vi "mod_Quantize BPSK symbols.vi"(0 "input data":dbl[](array[numeric]), 5 "quantization bits":i32=1, 11 "error in (no error)":errorcluster) -> (4 "output data":i32[](array[numeric]), 15 "error out":errorcluster)   [LabVIEW 2020, in "niDMT.lvlib"]
uses:
  <vilib>/addons/Modulation/niDMT.lvlib
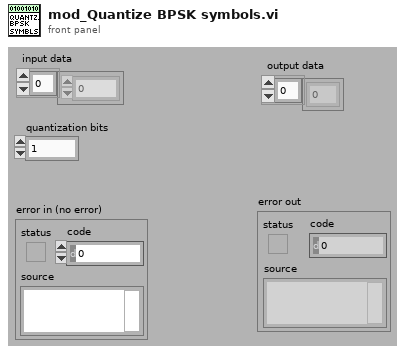
[diagram p1: front panel]
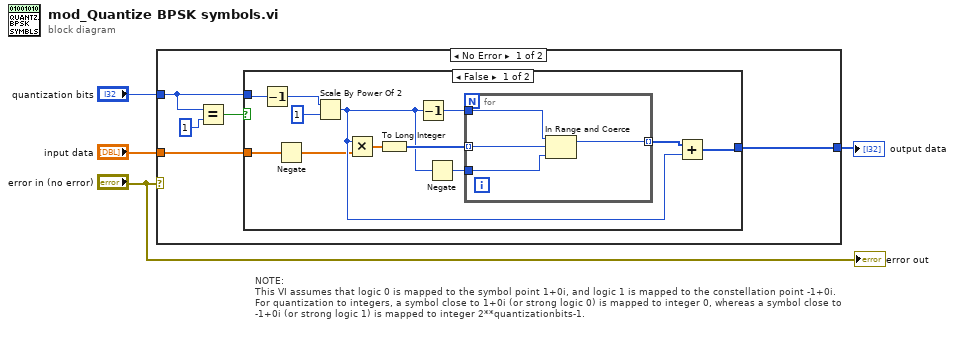
[diagram p0: block diagram]
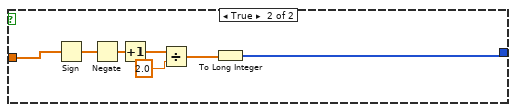
[diagram p2: hidden frame]
diagram:
  # "NOTE: \nThis VI assumes that logic 0 is mapped to the symbol point 1+0i, and logic 1 is mapped to the constellation point -1+0i.\nFor quantization to integers, a symbol close to 1+0i (or strong logic 0) is mapped to integer 0, whereas a symbol close to\n-1+0i (or strong logic 1) is mapped to integer 2**quantizationbits-1."
  n1 = case shown="No Error" "error in (no error)" {
    tunnel: "quantization bits" -> [w7 _]
    tunnel: "input data" -> [w9 _]
    tunnel: [w8 _] -> w1
    frame No Error {
      n2 = Equal?(x=w7, y=1) -> (x = y?=w5:bool)
      n3 = case shown="False" w5 {
        tunnel: w7 -> [w19 _]
        tunnel: w9 -> [w21 w32]
        tunnel: [w11 w31] -> w8
        frame False {
          n4 = Decrement(x=w19) -> (x-1=w18:i32)
          n5 = Negate(x=w21) -> (-x=w10:dbl[])
          n6 = Scale By Power Of 2(n=w18, x=1) -> (x*2^n=w12:i32)
          n7 = Multiply(x=w12, y=w10) -> (x*y=w17:dbl[])
          n8 = To Long Integer(number=w17) -> (32bit integer=w16:i32[])
          n9 = Decrement(x=w12) -> (x-1=w15:i32)
          n10 = Negate(x=w12) -> (-x=w14:i32)
          n11 = for {
            tunnel: w16 -> [w25] mode=indexing
            tunnel: w15 -> [w24]
            tunnel: w14 -> [w23]
            tunnel: [w22] -> w13 mode=indexing
            n12 = In Range and Coerce(upper limit=w24, x=w25, lower limit=w23) -> (coerced(x)=w22:i32)  [unwired: 1 out]
          }
          n13 = Add(x=w13, y=w12) -> (x+y=w11:i32[])
        }
        frame True {
          n14 = Sign(1:w32) -> (0:w30:dbl[])
          n15 = Negate(x=w30) -> (-x=w28:dbl[])
          n16 = Increment(x=w28) -> (x+1=w26:dbl[])
          n17 = Divide(x=w26, y=2.0) -> (x/y=w27:dbl[])
          n18 = To Long Integer(number=w27) -> (32bit integer=w31:i32[])
        }
      }
    }
    frame Error {
    }
  }
  "output data" <- w1
  "error out" <- "error in (no error)"
